vi "ParkField.vi"(2 "error in (no error)":errorcluster, 4 "Park?":bool) -> (0 "error out":errorcluster)   [LabVIEW 2020]
uses:
  Globals and TypeDefs/Global Varibal Control.vi
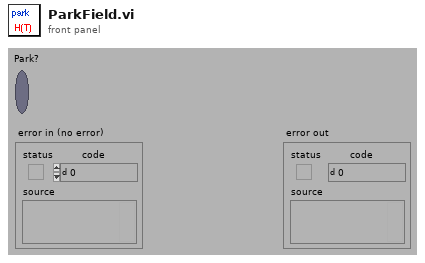
[diagram p1: front panel]
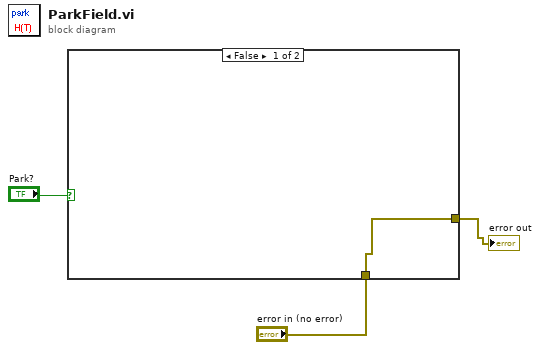
[diagram p0: block diagram]
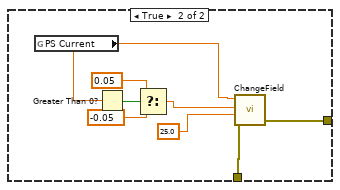
[diagram p2: hidden frame]
diagram:
  n1 = case shown="False" "Park?" {
    tunnel: "error in (no error)" -> [w4 w6]
    tunnel: [w4 w5] -> w1
    frame False {
    }
    frame True {
      n2 = global read "Global Varibal Control.vi" "PS Current"() -> (w8:dbl)
      n3 = Greater Than 0?(x=w8) -> (x > 0?=w12:bool)
      n4 = Select(t=0.05, s=w12, f=-0.05) -> (s? t:f=w11:dbl)
      n5 = call "ChangeField.vi"("Starting Field (T)"=w8, "Desired Field (T)"=w11, "Magnet System"=25.0 ("SweepRate (T/min)"), "error in (no error)"=w6) -> ("error out"=w5:errorcluster)  [unwired: 2 in, 2 out]
    }
  }
  "error out" <- w1
